vi "Create Measurement.vi"(8 "error in":errorcluster) -> (0 "error out":errorcluster, 3 "gRPCid out":T1)   [LabVIEW 2021, in "Measurement Client Template.lvlib"]
doc: "Create client for the measurement service and complete metadata registration."
uses:
  Measurement Client Template.lvlib
  <vilib>/gRPC/LabVIEW gRPC Library/Shared/grpcId.ctl
  <vilib>/gRPC/Generated APIs/ni/measurementlink/discovery/v1/RPC Messages/ni_measurementlink_discovery_v1_ResolveServiceRequest.ctl
  controls/Measurement Results.ctl
  controls/Measurement Configuration.ctl
  <vilib>/Plug-In SDKs/Clients/Discovery V1/NI Discovery V1 Client.lvlib
  <vilib>/gRPC/Generated APIs/ni/measurementlink/discovery/v1/ni.measurementlink.discovery.v1.api.lvlib
  <vilib>/gRPC/LabVIEW gRPC Library/grpc-lvsupport-release.lvlib
  <vilib>/gRPC/Generated APIs/ni/measurementlink/measurement/v2/Measurement Service Client V2/Measurement Service Client V2.lvlib
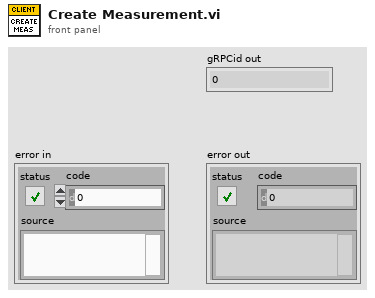
[diagram p1: front panel]
types:
  T1 = typedef "grpc-lvsupport-release.lvlib/grpcId.ctl" = u64
  T2 = typedef "Measurement Client Template.lvlib/Measurement Configuration.ctl" = cluster{"Boolean":bool}
  T3 = typedef "Measurement Client Template.lvlib/Measurement Results.ctl" = cluster{"Boolean":bool}
  T4 = typedef "ni.measurementlink.discovery.v1.api.lvlib/ni_measurementlink_discovery_v1_ResolveServiceRequest.ctl" = cluster{"provided_interface":string, "service_class":string, "deployment_target":string, "version":string}
  T5 = typedef "ni.measurementlink.discovery.v1.api.lvlib/ni_measurementlink_discovery_v1_ServiceLocation.ctl" = cluster{"location":string, "insecure_port":string, "ssl_authenticated_port":string}
  T6 = typedef "grpc-lvsupport-release.lvlib/Enum Metadata.ctl" = cluster{"Version":i32, "Name":string, "Type Url":string, "Enum Values":string, "Allow Alias":bool}
  T7 = typedef "grpc-lvsupport-release.lvlib/Message Metadata.ctl" = cluster{"Version":i32, "Name":string, "Type Url":string, "Elements":T8[], "Has Oneof":bool}
  T8 = typedef "grpc-lvsupport-release.lvlib/Message Element Metadata.ctl" = cluster{"Field Name":string, "Embedded Message Name":string, "Protobuf Index":i32, "MessageElementType":T9, "Repeated":bool, "Is in Oneof":bool, "Oneof Container Name":string}
  T9 = typedef "grpc-lvsupport-release.lvlib/Message Element Type.ctl" = enum32{"Int32Value", "FloatValue", "DoubleValue", "BoolValue", "StringValue", "MessageValue", "Int64Value", "UInt32Value", "UInt64Value", "EnumValue", "Bytes", "Fixed64", "Fixed32", "SFixed64", "SFixed32", "SInt64", "SInt32"}
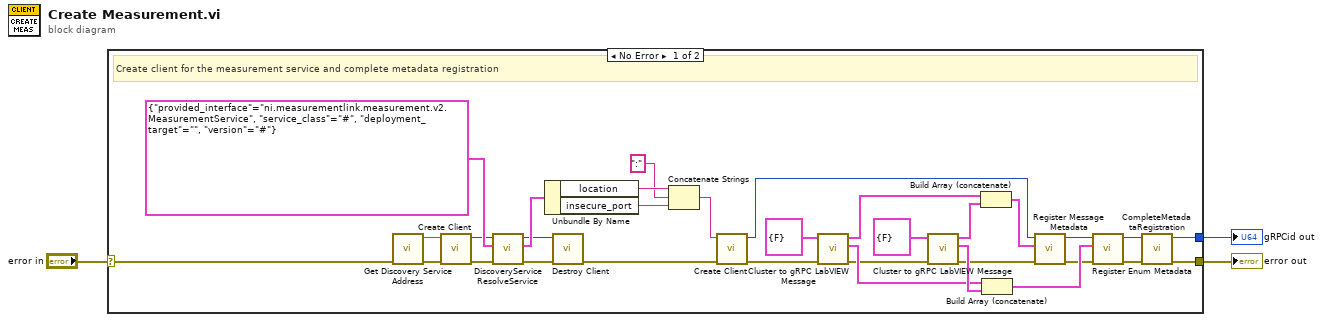
[diagram p0: block diagram]
diagram:
  n1 = case shown="No Error" "error in" {
    selector: "error in" -> [w32 w36]
    tunnel: [w16 w36] -> w2
    tunnel: [w15 _] -> w1
    frame No Error {
      # "Create client for the measurement service and complete metadata registration"
      n2 = call <vilib>:"Get Discovery Service Address.vi"("error in"=w32) -> ("error out"=w33:errorcluster, "address"=w34:string)  [unwired: 9 in]
      n3 = call <vilib>:"Create Client.vi"("error in"=w33, "address"=w34) -> ("error out"=w31:errorcluster, "gRPC ID Out"=w7:T1)  [unwired: 8 in]
      n4 = call <vilib>:"DiscoveryService ResolveService.vi"("error in"=w31, "Request Data"=T4 {"provided_interface"="ni.measurementlink.measurement.v2.MeasurementService", "service_class"="#", "deployment_target"="", "version"="#"} ("resolve service request data"), "gRPC ID"=w7) -> ("error out"=w28:errorcluster, "Response Data"=w30:T5, "gRPC ID out"=w29:T1)  [unwired: 6 in]
      n5 = Unbundle By Name(w30) -> ("location"=w12:string, "insecure_port"=w11:string)
      n6 = call <vilib>:"Destroy Client.vi"("error in"=w28, "gRPC ID"=w29) -> ("error out"=w27:errorcluster)  [unwired: 9 in]
      n7 = Concatenate Strings(w12, ":" ("string"), w11) -> (w10:string)
      n8 = call <vilib>:"Create Client.vi"("error in"=w27, "address"=w10) -> ("error out"=w14:errorcluster, "gRPC ID Out"=w21:T1)  [unwired: 8 in]
      n9 = call <vilib>:"Cluster to gRPC LabVIEW Message.vi"("error in"=w14, "Cluster"=T2 {"Boolean"=FALSE} ("measurement configuration")) -> ("error out"=w13:errorcluster, "gRPC Enum Metadata out"=w25:T6[], "gRPC Message Metadata []"=w20:T7[])  [unwired: 7 in]
      n10 = call <vilib>:"Cluster to gRPC LabVIEW Message.vi"("error in"=w13, "Cluster"=T3 {"Boolean"=FALSE} ("measurement results")) -> ("error out"=w17:errorcluster, "gRPC Enum Metadata out"=w26:T6[], "gRPC Message Metadata []"=w18:T7[])  [unwired: 7 in]
      n11 = Build Array (concatenate)(w20, w18) -> (w19:T7[])
      n12 = Build Array (concatenate)(w25, w26) -> (w24:T6[])
      n13 = call <vilib>:"Register Message Metadata.vi"("error in"=w17, "Messages"=w19, "gRPCid in"=w21) -> ("error out"=w22:errorcluster, "gRPCid out"=w35:T1)  [unwired: 7 in]
      n14 = call <vilib>:"Register Enum Metadata.vi"("error in"=w22, "Enum Metadata"=w24, "gRPCid in"=w35) -> ("error out"=w23:errorcluster, "gRPCid out"=w4:T1)  [unwired: 7 in]
      n15 = call <vilib>:"CompleteMetadataRegistration.vi"("error in"=w23, "gRPC ID in"=w4) -> ("error out"=w16:errorcluster, "gRPC ID Out"=w15:T1)  [unwired: 8 in]
    }
    frame Error {
      # "Pass"
    }
  }
  "error out" <- w2
  "gRPCid out" <- w1
